vi "add_frequency.vi"(0 "Freq value":dbl, 9 "Add Button":bool) -> ()   [LabVIEW 2016]
panel:
  out "output array":i32[](array[numeric])
  in  "Array":i32[](array[numeric])
  in  "Stop":bool
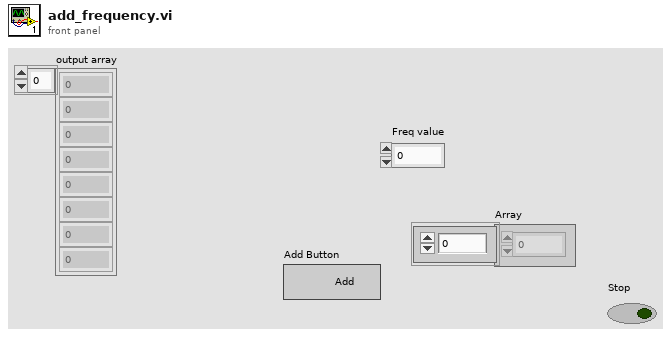
[diagram p1: front panel]
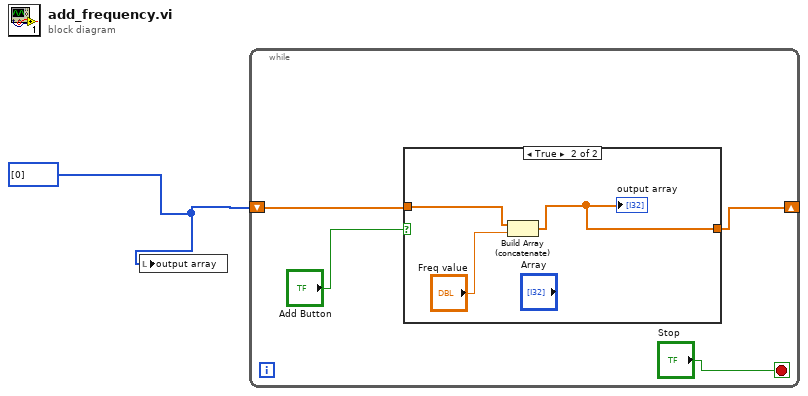
[diagram p0: block diagram]
diagram:
  w1 = i32[] [0]
  n1 = local write "output array"(w1) -> ()
  n2 = while {
    shift-right: [w2] -> _
    shift-left: w1 -> [w3]
    stop <- "Stop" stop-if-true
    n3 = case shown="True" "Add Button" {
      tunnel: w3 -> [w6 w8]
      tunnel: [w6 w7] -> w2
      frame False {
      }
      frame True {
        n4 = Build Array (concatenate)(w8, "Freq value") -> (w7:dbl[])
        "output array" <- w7
      }
    }
  }
